vi "Actor Core.vi"(8 "error in":errorcluster, 11 "Cooler in":refnum<class "Cooler.lvclass">) -> (0 "error out":errorcluster, 3 "Actor out":refnum<class "Actor.lvclass">)   [LabVIEW 2012, in "Cooler.lvlib" / "Cooler.lvclass"]
doc: "(<B>Filename</B>: Actor Framework.lvlib:Actor.lvclass:Actor Core.vi)\n\nReceives messages to the actor, reacts to them, and initiates any error handling that may shut the actor down.\n\nDescendant classes may override this VI to append parallel tasks for the actor to complete while it handles messages. Overrides use the Call Parent Method node."
uses:
  Cooler.lvclass
  <vilib>/ActorFramework/Actor/Actor.lvclass
  Dual Controller/Dual Fan/Dual Fan.lvclass
  Water Level/Water Level.lvclass
  <vilib>/ActorFramework/Actor/Actor.lvclass/Actor.ctl
  <vilib>/ActorFramework/Message Enqueuer/Message Enqueuer.lvclass/Message Enqueuer.ctl
  Cooler.lvclass/Cooler.ctl
  Level Controller/Level Controller/Level Controller.lvclass
  <vilib>/ActorFramework/Message Enqueuer/Init from Existing Queue.vi
  <vilib>/ActorFramework/Message Enqueuer/Message Enqueuer.lvclass
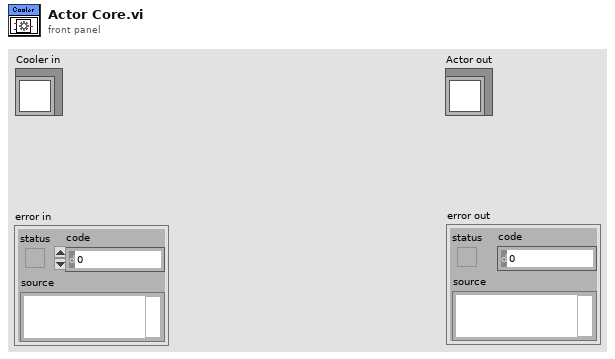
[diagram p1: front panel]
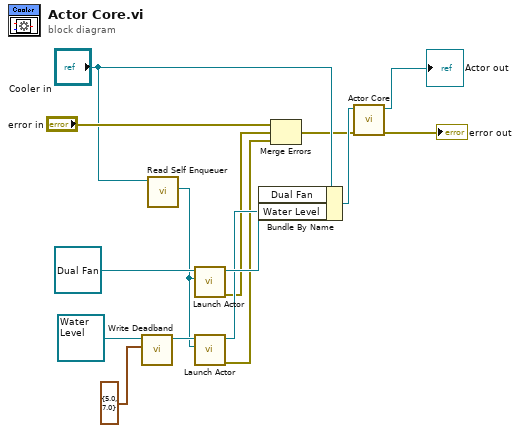
[diagram p0: block diagram]
diagram:
  n1 = call "Write Deadband.vi"("Deadband"=cluster{"LO":dbl, "HI":dbl} {"LO"=5.0, "HI"=7.0}, "Level Controller in"=refnum<class "Water Level.lvclass"> refnum ("Water Level.lvclass")) -> ("Level Controller out"=w10:refnum<class "Water Level.lvclass">)  [unwired: 8 in, 1 out]
  n2 = call <vilib>:"Read Self Enqueuer.vi"("Actor"="Cooler in") -> ("Self Enqueuer"=w1:refnum<class "Message Enqueuer.lvclass">)  [unwired: 10 in]
  n3 = call <vilib>:"Launch Actor.vi"("Actor-to-Caller Enqueuer"=w1, "Actor"=refnum<class "Dual Fan.lvclass"> refnum ("Dual Fan.lvlib:Dual Fan.lvclass")) -> ("error out"=w3:errorcluster, "Caller-To-Actor Enqueuer"=w6:refnum<class "Message Enqueuer.lvclass">)  [unwired: 8 in]
  n4 = call <vilib>:"Launch Actor.vi"("Actor-to-Caller Enqueuer"=w1, "Actor"=w10) -> ("error out"=w2:errorcluster, "Caller-To-Actor Enqueuer"=w5:refnum<class "Message Enqueuer.lvclass">)  [unwired: 8 in]
  n5 = Bundle By Name(cluster="Cooler in", "Dual Fan"=w6, "Water Level"=w5) -> (w7:refnum<class "Cooler.lvclass">)
  n6 = Merge Errors("error in", w3, w2) -> (w4:errorcluster)
  n7 = call-parent "Actor Core.vi"("error in"=w4, "Timed Loop Controller in"=w7) -> ("error out"=→"error out":errorcluster, "Actor out"=→"Actor out":refnum<class "Actor.lvclass">)  [unwired: 8 in]
